vi "LWXPS_ElapsedTimeGet.vi"(0 "XPS Reference IN":refnum<k24>, 11 "LabVIEW error IN":errorcluster) -> (4 "XPS Reference OUT":refnum<k24>, 6 "Returned error code":i32, 8 "Elapsed Time":dbl, 10 "XPS Error String":string, 15 "LabVIEW error OUT":errorcluster)   [LabVIEW 2013]
uses:
  Newport.XPS.CommandInterface
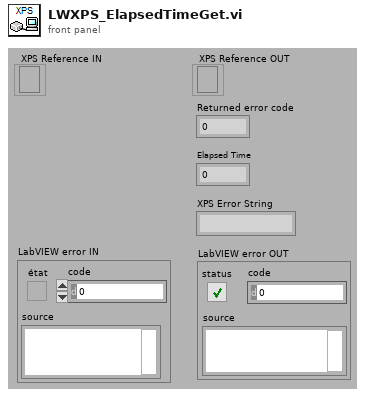
[diagram p1: front panel]
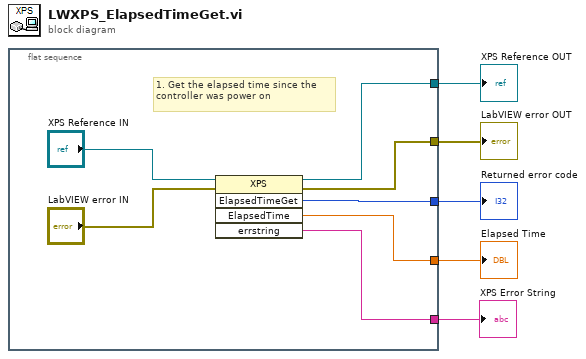
[diagram p0: block diagram]
diagram:
  n1 = flat-sequence {
    tunnel: [w9] -> w5
    tunnel: [w12] -> w4
    tunnel: [w8] -> w1
    tunnel: [w7] -> w3
    tunnel: [w6] -> w2
    frame #0 {
      # "1. Get the elapsed time since the controller was power on"
      n2 = invoke class="XPS" method="ElapsedTimeGet"(reference="XPS Reference IN", error in="LabVIEW error IN") -> (reference out=w9:refnum<k24>, error out=w12:errorcluster, "ElapsedTimeGet"=w8:i32, "ElapsedTime"=w6:dbl, "errstring"=w7:string)  [unwired: 3 in]
    }
  }
  "XPS Reference OUT" <- w5
  "LabVIEW error OUT" <- w4
  "XPS Error String" <- w3
  "Elapsed Time" <- w2
  "Returned error code" <- w1
